vi "Close.vi"(8 "error in (no error)":errorcluster {"code" format="Error %.0f"}, 11 "VIDoc Printer In":refnum<class "VIDoc Printer.lvclass">) -> (0 "error out":errorcluster {"code" format="Error %.0f"})   [LabVIEW 2023, in "VIDoc Printer.lvlib" / "VIDoc Printer.lvclass"]
doc: "Close the Report. Closes references, connections or anything else that needs to be closed at end of reporting."
uses:
  VIDoc Printer.lvclass
  VIDoc Printer.lvclass/VIDoc Printer.ctl
  UI Interaction/UI Interaction.lvclass
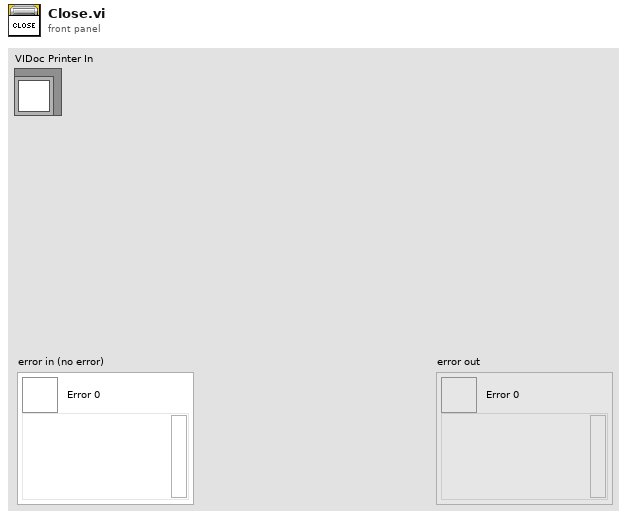
[diagram p1: front panel]
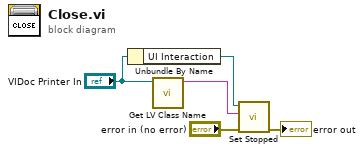
[diagram p0: block diagram]
diagram:
  n1 = Unbundle By Name("VIDoc Printer In") -> ("UI Interaction"=w3:refnum<class "UI Interaction.lvclass">)
  n2 = call <vilib>:"Get LV Class Name.vi"("object"="VIDoc Printer In") -> ("class name"=w1:string)  [unwired: 9 in, 1 out]
  n3 = call-dynamic "Set Stopped.vi"("error in (no error)"="error in (no error)", "Process"=w1, "UI Interaction in"=w3) -> ("error out"=→"error out":errorcluster)  [unwired: 7 in, 1 out]
